vi "Data View - Parse Test Plan (SubVI).vi"(11 "data":T1(array[cluster])) -> (3 "Test Plan":string[](array[string]))   [LabVIEW 2019]
uses:
  <userlib>/_OpenG.lib/array/array.llb/Remove Duplicates from 1D Array (String)__ogtk.vi
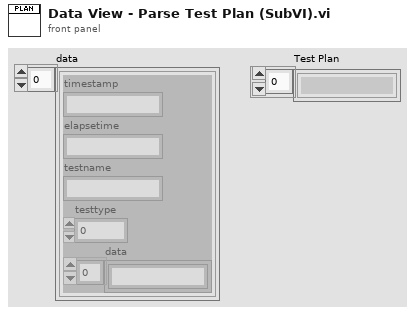
[diagram p1: front panel]
types:
  T1 = cluster{"timestamp":string, "elapsetime":string, "testname":string, "testtype":u16, "data":string[]}[]
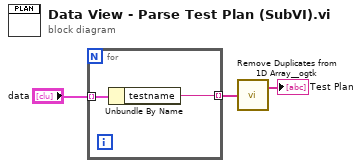
[diagram p0: block diagram]
diagram:
  n1 = for {
    tunnel: "data" -> [w5] mode=indexing
    tunnel: [w4] -> w2 mode=indexing
    n2 = Unbundle By Name(w5) -> ("testname"=w4:string)
  }
  n3 = call-poly <userlib>:"Remove Duplicates from 1D Array__ogtk.vi"("Input Array"=w2) -> ("Output Array"=→"Test Plan":string[])  [unwired: 1 out]
